vi "Pre Launch Init.vi"(11 "DAQ DI in":refnum<class "DAQ DI.lvclass">) -> (0 "error out":errorcluster, 3 "DAQ DI out":refnum<class "DAQ DI.lvclass">)   [LabVIEW 2020, in "DAQ DI.lvlib" / "DAQ DI.lvclass"]
doc: "<p>(<strong>Filename</strong>: <span class=\"dnl\">Actor Framework.lvlib:Actor.lvclass:Pre Launch Init.vi</span>)</p>\n<p>Defines behavior that occurs after the <a href=\"nihelplauncher://docs/csh?context=lvcore_lvcomm_af_launch_nested_actor\">Launch Nested Actor</a> method is invoked but before the actor's Actor Core method begins running.</p>\n<p>By default, this method does nothing. A descendant class may override it to define behavior.</p>"
uses:
  DAQ DI.lvclass
  DAQ DI.lvclass/DAQ DI.ctl
  <vilib>/ActorFramework/Actor/Actor.lvclass
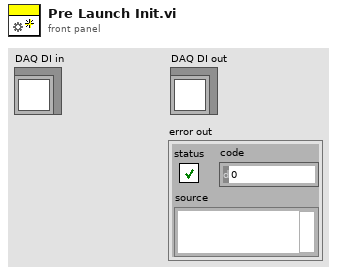
[diagram p1: front panel]
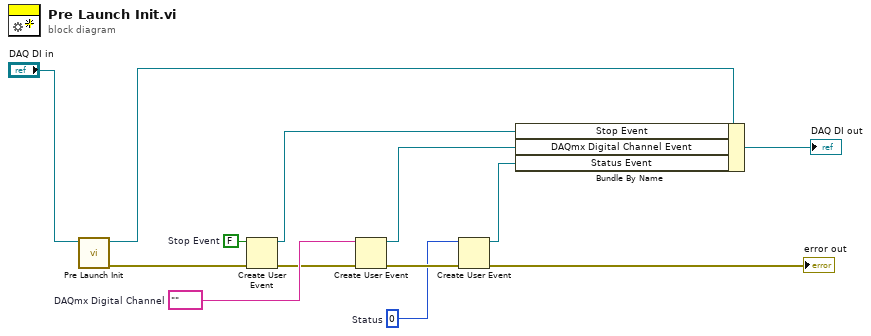
[diagram p0: block diagram]
diagram:
  w1 = u8 0  # Status
  w10 = FALSE  # Stop Event
  w12 = tag ""  # DAQmx Digital Channel
  n1 = call-parent "Pre Launch Init.vi"("Actor in"="DAQ DI in") -> ("error out"=w5:errorcluster, "Actor out"=w7:refnum<class "DAQ DI.lvclass">)  [unwired: 9 in]
  n2 = Create User Event(user event datatype=w10, error in=w5) -> (user event=w8:refnum<user-event>, error out=w9:errorcluster)
  n3 = Create User Event(user event datatype=w12, error in=w9) -> (user event=w11:refnum<user-event>, error out=w4:errorcluster)
  n4 = Create User Event(user event datatype=w1, error in=w4) -> (user event=w2:refnum<user-event>, error out=→"error out":errorcluster)
  n5 = Bundle By Name(cluster=w7, "Stop Event"=w8, "DAQmx Digital Channel Event"=w11, "Status Event"=w2) -> (→"DAQ DI out":refnum<class "DAQ DI.lvclass">)
